vi "SetActiveAlarms.vi"(8 "error in (no error)":errorcluster, 10 "ActiveAlarms":T2[](array[typedef]), 11 "config in":T1) -> (0 "error out":errorcluster, 3 "config out":T1)   [LabVIEW 2017, in "TrendAlarm.lvlib"]
uses:
  <vilib>/addons/InsightCM/Devices/Shared/Common/TrendAlarm/TrendAlarm.lvlib
  <vilib>/addons/InsightCM/MessageBus/Base/controls/TrendAlarmInstance.ctl
  <vilib>/addons/InsightCM/MessageBus/Base/controls/TrendAlarmTransition.ctl
  <vilib>/addons/InsightCM/Devices/Shared/Common/TrendAlarm/controls/config.ctl
  <vilib>/addons/InsightCM/Devices/Shared/Common/TrendAlarm/controls/TransitionCache.ctl
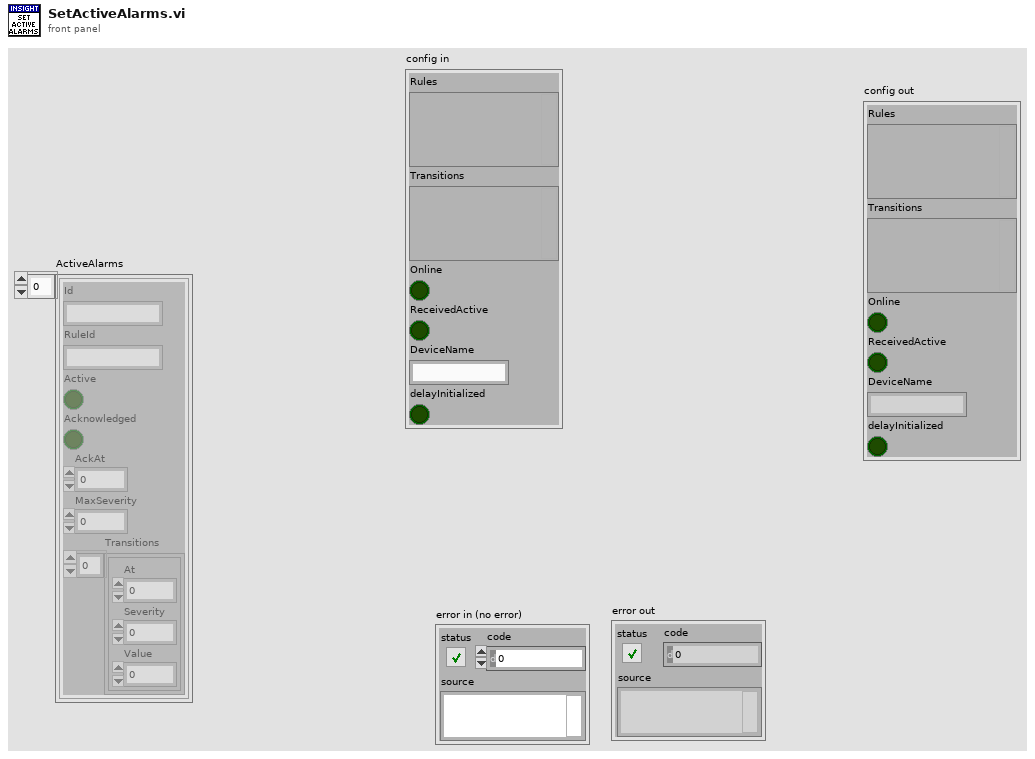
[diagram p1: front panel]
types:
  T1 = typedef "TrendAlarm.lvlib/config.ctl" = cluster{"Rules":variant, "Transitions":variant, "Online":bool, "ReceivedActive":bool, "DeviceName":string, "delayInitialized":bool}
  T2 = typedef "TrendAlarmInstance.ctl" = cluster{"Id":string, "RuleId":string, "Active":bool, "Acknowledged":bool, "AckAt":i64, "MaxSeverity":i32, "Transitions":T3[]}
  T3 = typedef "TrendAlarmTransition.ctl" = cluster{"At":i64, "Severity":i32, "Value":dbl}
  T4 = typedef "TrendAlarm.lvlib/TransitionCache.ctl" = cluster{"RuleId":string, "MaxSeverity":i32, "LastTransition":T3, "OnTime":timestamp, "OffTime":timestamp}
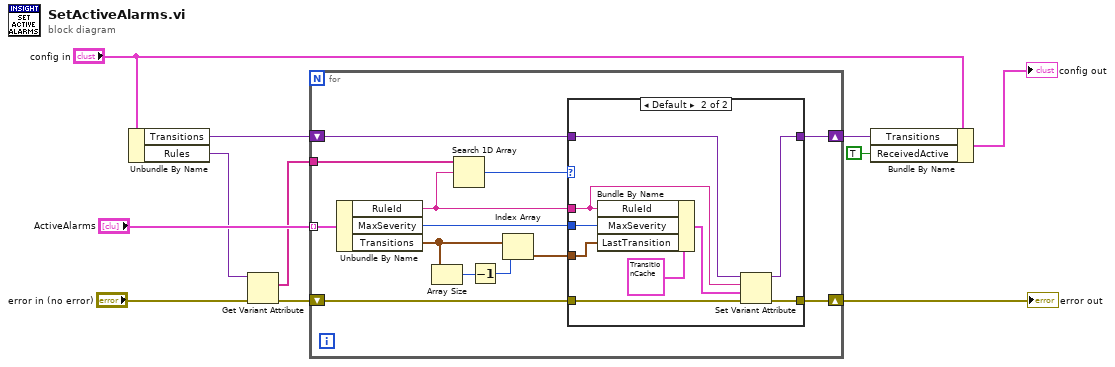
[diagram p0: block diagram]
diagram:
  n1 = Unbundle By Name("config in") -> ("Transitions"=w1:variant, "Rules"=w9:variant)
  n2 = Get Variant Attribute(Variant=w9, error in="error in (no error)") -> (names=w8:string[], error out=w7:errorcluster)  [unwired: 2 in, 2 out]
  n3 = for {
    tunnel: "ActiveAlarms" -> [w24] mode=indexing
    tunnel: w8 -> [w20]
    shift-right: [w17] -> w5
    shift-left: w1 -> [w18]
    shift-right: [w12] -> w2
    shift-left: w7 -> [w19]
    n4 = Unbundle By Name(w24) -> ("RuleId"=w14:string, "MaxSeverity"=w15:i32, "Transitions"=w21:T3[])
    n5 = Array Size(array=w21) -> (size(s)=w23:i32)
    n6 = Search 1D Array(1D array=w20, element=w14) -> (index of element=w13:i32)  [unwired: 1 in]
    n7 = Decrement(x=w23) -> (x-1=w22:i32)
    n8 = Index Array(array=w21, index=w22) -> (element=w16:T3)
    n9 = case shown="Default" w13 {
      tunnel: w19 -> [w25 w34]
      tunnel: w18 -> [w26 w33]
      tunnel: [w26 w32] -> w17
      tunnel: w16 -> [_ w31]
      tunnel: w15 -> [_ w30]
      tunnel: w14 -> [_ w27]
      tunnel: [w25 w28] -> w12
      frame -1 {
      }
      frame Default {
        n10 = Bundle By Name(cluster=T4 {"RuleId"="", "MaxSeverity"=0, "LastTransition"={"At"=0, "Severity"=0, "Value"=0.0}, "OnTime"=timestamp(0 s since 1904-01-01), "OffTime"=timestamp(0 s since 1904-01-01)} ("TransitionCache"), "RuleId"=w27, "MaxSeverity"=w30, "LastTransition"=w31) -> (w29:T4)
        n11 = Set Variant Attribute(Variant=w33, name=w27, value=w29, error in=w34) -> (Variant out=w32:variant, error out=w28:errorcluster)  [unwired: 1 out]
      }
    }
  }
  "error out" <- w2
  n12 = Bundle By Name(cluster="config in", "Transitions"=w5, "ReceivedActive"=TRUE) -> (→"config out":T1)
